vi "MoveAbsSingleAxis.vi"(6 "Wait":bool=TRUE, 8 "error in (no error)":errorcluster, 9 "Value":dbl format="%.2f", 10 "Axis":i32=1, 11 "OWIS_TANGO in":refnum<class "OWIS_TANGO.lvclass">) -> (0 "error out":errorcluster, 3 "OWIS_TANGO out":refnum<class "OWIS_TANGO.lvclass">)   [LabVIEW 2020, in "OWIS_TANGO.lvclass"]
uses:
  OWIS_TANGO.lvclass
  OWIS_TANGO.lvclass/OWIS_TANGO.ctl
  tango-binding-3.0.0-for-labview-2015-windows-x86/vis/tango_vi.llb/_TangoWriteDoubleScalarAttribute.vi
  tango-binding-3.0.0-for-labview-2014-windows-x64/vis/tango_vi.llb/tango.lvlib
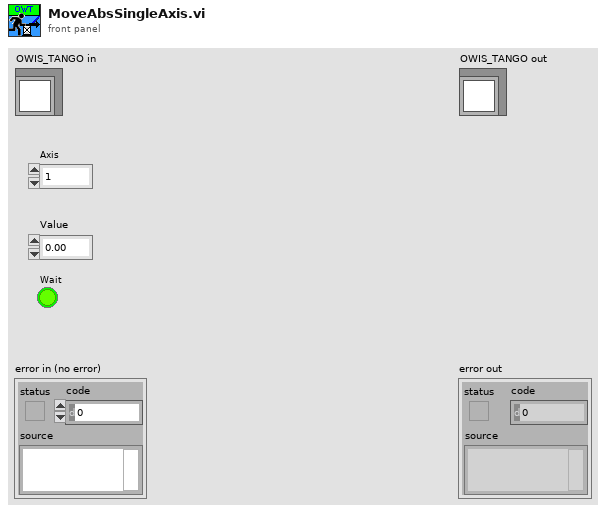
[diagram p1: front panel]
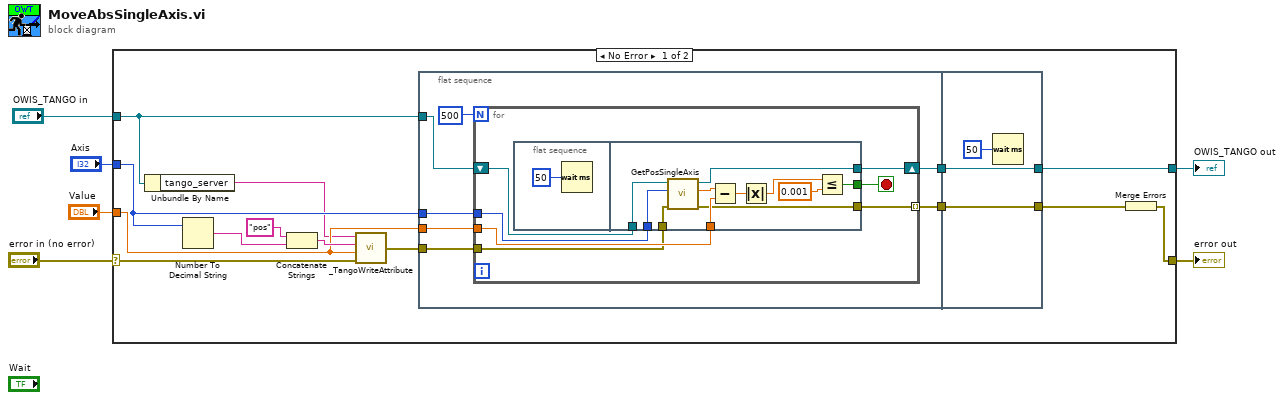
[diagram p0: block diagram]
diagram:
  n1 = case shown="No Error" "error in (no error)" {
    selector: "error in (no error)" -> [w15 w50]
    tunnel: "OWIS_TANGO in" -> [w10 w51]
    tunnel: [w20 w51] -> w4
    tunnel: [w12 w50] -> w3
    tunnel: "Value" -> [w11 _]
    tunnel: "Axis" -> [w16 _]
    frame No Error {
      n2 = Unbundle By Name(w10) -> ("tango_server"=w9:string)
      n3 = Number To Decimal String(number=w16) -> (decimal integer string=w18:string)  [unwired: 1 in]
      n4 = Concatenate Strings("pos" ("attribute name"), w18) -> (w17:string)
      n5 = call-poly "_TangoWriteAttribute.vi"("error in"=w15, "value"=w11, "attribute name"=w17, "device name"=w9) -> ("error out"=w14:errorcluster)
      n6 = flat-sequence {
        tunnel: w16 -> [w25]
        tunnel: w14 -> [w24]
        tunnel: w11 -> [w22]
        tunnel: w10 -> [w21]
        tunnel: [w27] -> w8
        tunnel: [w23] -> w7
        tunnel: w8 -> [w49]
        tunnel: w7 -> [w48]
        tunnel: [w49] -> w20
        tunnel: [w48] -> w13
        frame #0 {
          n7 = for {
            N: 500 -> [_]
            tunnel: w22 -> [w34]
            tunnel: w25 -> [w33]
            shift-right: [w31] -> w27
            shift-left: w21 -> [w32]
            tunnel: w24 -> [w29]
            tunnel: [w28] -> w23 mode=indexing
            stop <- w30 stop-if-true
            n8 = flat-sequence {
              tunnel: [w43] -> w30
              tunnel: w34 -> [w41]
              tunnel: w33 -> [w40]
              tunnel: w32 -> [w39]
              tunnel: [w38] -> w31
              tunnel: w29 -> [w37]
              tunnel: [w36] -> w28
              frame #0 {
                n9 = Wait (ms)(milliseconds to wait=u32 50) -> ()  [unwired: 1 out]
              }
              frame #1 {
                n10 = call-dynamic "GetPosSingleAxis.vi"("error in (no error)"=w37, "Axis"=w40, "OWIS_TANGO in"=w39) -> ("error out"=w36:errorcluster, "Pos"=w42:dbl, "OWIS_TANGO out"=w38:refnum<class "OWIS_TANGO.lvclass">)  [unwired: 6 in]
                n11 = Subtract(x=w42, y=w41) -> (x-y=w46:dbl)
                n12 = Absolute Value(x=w46) -> (abs(x)=w45:dbl)
                n13 = Less Or Equal?(x=w45, y=0.001) -> (x <= y?=w43:bool)
              }
            }
          }
        }
        frame #1 {
          n14 = Wait (ms)(milliseconds to wait=u32 50) -> ()  [unwired: 1 out]
        }
      }
      n15 = Merge Errors(w13) -> (w12:errorcluster)
    }
    frame Error {
    }
  }
  "error out" <- w3
  "OWIS_TANGO out" <- w4
